vi "Select Device Dialog.vi"(7 "Filter Type":T1=enum."Product Name", 8 "error in (no error)":errorcluster, 10 "Filter Names":string[](array[string]), 11 "Item Ref in":T2 format="%.0x") -> (0 "error out":errorcluster, 1 "Cancelled?":bool, 2 "Selected Alias":string, 3 "Item Ref out":T2=18446744073709551615 format="%.0x")   [LabVIEW 2015, in "NIVS Hardware Discovery.lvlib"]
uses:
  NIVS Hardware Discovery.lvlib
  <vilib>/NI Veristand/Custom Device API/Custom Device Item Ref.ctl
  Types/Filter Type.ctl
  <vilib>/NI Veristand/Custom Device API/Custom Device API.lvlib
panel:
  in  "Cancel":bool
  in  "Use Selected":bool
  in  "Refresh":bool
  in  "Compatible Devices":u16(ring)
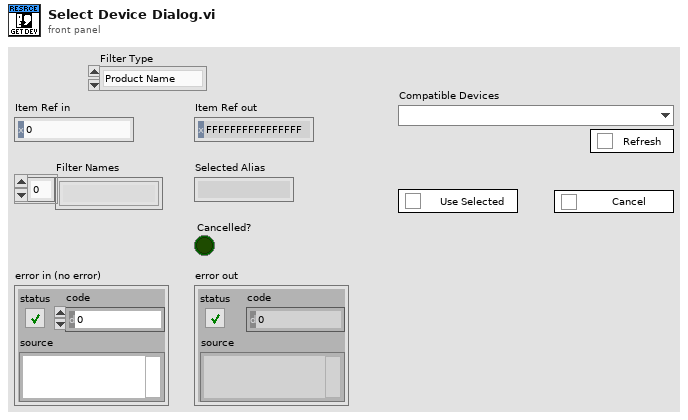
[diagram p1: front panel]
types:
  T1 = typedef "NIVS Hardware Discovery.lvlib/Filter Type.ctl" = enum16{"Device Category", "Product Name", "Ethernet", "XNET", "VISA", "FPGA", "EtherCAT Master", "DAQmx"}
  T2 = typedef "Custom Device API.lvlib/Custom Device Item Ref.ctl" = u64
  T3 = enum32{"Invalid", "Standard", "Closed", "Hidden", "Minimized", "Maximized"}
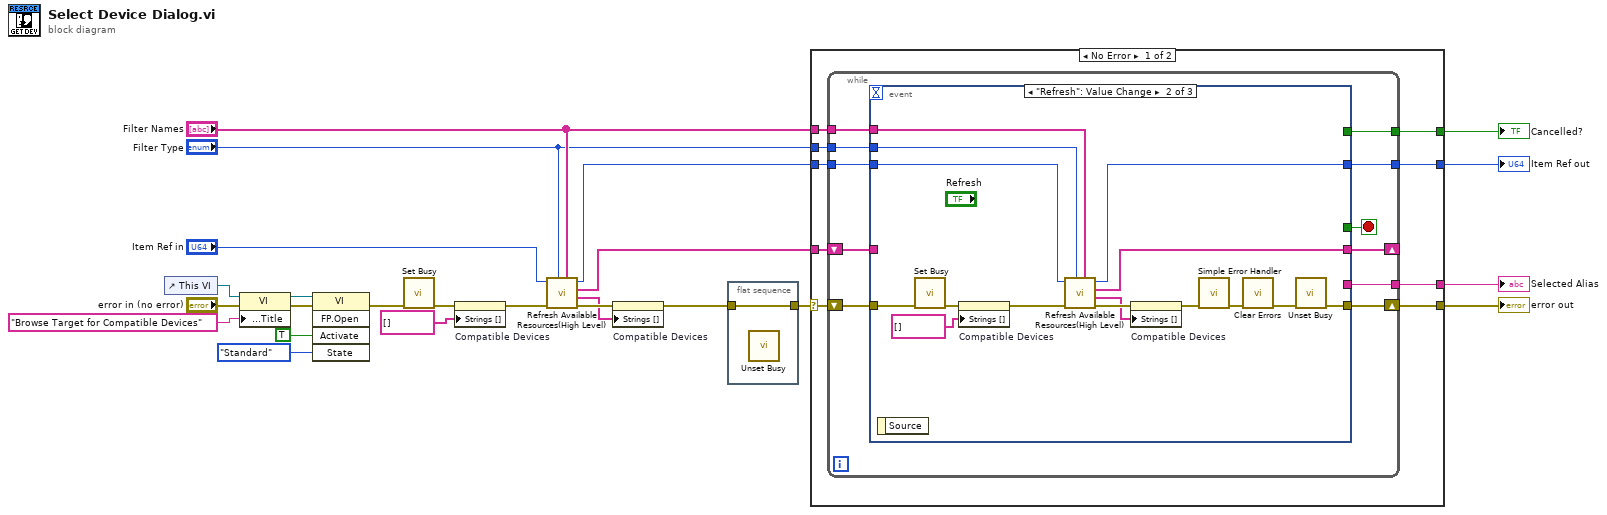
[diagram p0: block diagram]
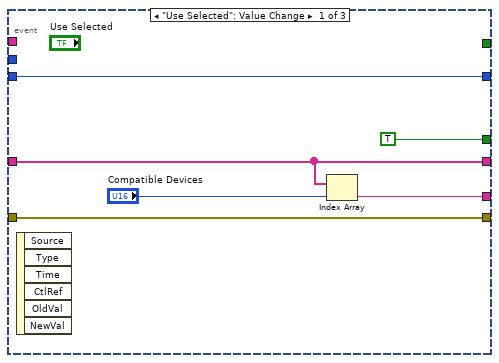
[diagram p2: hidden frame]
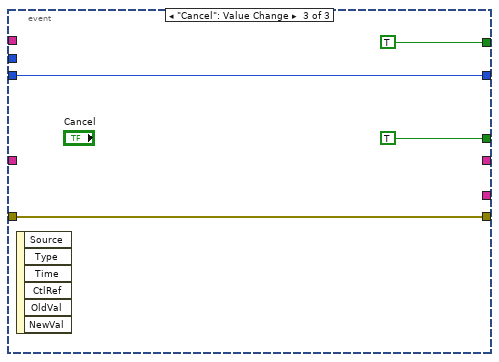
[diagram p3: hidden frame]
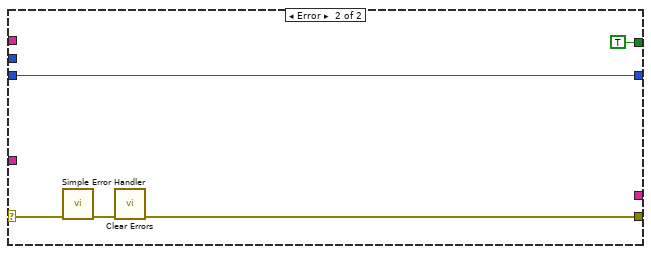
[diagram p4: hidden frame]
diagram:
  n1 = control-ref of="This VI"() -> (w16:refnum<vi>)
  n2 = property class="VI"(reference=w16, error in="error in (no error)", "Front Panel.Title"="Browse Target for Compatible Devices" ("Front Panel Window:Title")) -> (reference out=w14:refnum<vi>, error out=w13:errorcluster)
  n3 = invoke class="VI" method="FP.Open"(reference=w14, error in=w13, "Activate"=TRUE ("Activate?"), "State"=T3."Standard") -> (error out=w4:errorcluster)  [unwired: 1 in, 4 out]
  n4 = call <vilib>:"Set Busy.vi"("error in (no error)"=w4) -> ("error out"=w3:errorcluster)  [unwired: 9 in, 1 out]
  n5 = property on="Compatible Devices" class="Ring (strict)"(error in=w3, "Strings []"=string[] []) -> (error out=w6:errorcluster)  [unwired: 1 in, 1 out]
  n6 = call "Refresh Available Resources(High Level).vi"("Filter Names"="Filter Names", "Filter Type"="Filter Type", "error in (no error)"=w6, "Section Ref in"="Item Ref in") -> ("error out"=w9:errorcluster, "Name and Alias"=w7:string[], "Aliases"=w8:string[], "Section Ref out"=w10:T2)  [unwired: 4 in]
  n7 = property on="Compatible Devices" class="Ring (strict)"(error in=w9, "Strings []"=w7) -> (error out=w1:errorcluster)  [unwired: 1 in, 1 out]
  n8 = flat-sequence {
    tunnel: [w25] -> w2
    tunnel: w1 -> [w25]
    frame #0 {
      n9 = call <vilib>:"Unset Busy.vi"() -> ()  [unwired: 11 in, 1 out]
    }
  }
  n10 = case shown="No Error" w2 {
    selector: w2 -> [w26 w75]
    tunnel: [w34 w72] -> w23
    tunnel: [w33 _] -> w22
    tunnel: "Filter Names" -> [w32 _]
    tunnel: [w31 TRUE] -> w20
    tunnel: [w30 w73] -> w17
    tunnel: "Filter Type" -> [w29 _]
    tunnel: w10 -> [w28 w72]
    tunnel: w8 -> [w27 _]
    frame No Error {
      n11 = while {
        shift-right: [w41] -> w30
        shift-left: w26 -> [w42]
        tunnel: [w44] -> w33
        tunnel: w28 -> [w40]
        shift-right: [w38] -> _
        shift-left: w27 -> [w45]
        tunnel: w32 -> [w39]
        tunnel: [w37] -> w31
        tunnel: [w36] -> w34
        tunnel: w29 -> [w35]
        stop <- w43 stop-if-true
        n12 = event shown="[1] \"Refresh\": Value Change" {
          selector: _ -> [_ _ _]
          dyn-events: _ -> [_ _ _]
          timeout: _ -> [_ _ _]
          tunnel: w45 -> [w47 _ _]
          tunnel: [w50 _ _] -> w44
          tunnel: [TRUE _ TRUE] -> w43
          tunnel: w42 -> [w48 w55 w67]
          tunnel: [w48 w52 w67] -> w41
          tunnel: w40 -> [w46 w66 w68]
          tunnel: w39 -> [_ w62 _]
          tunnel: [w47 w61 _] -> w38
          tunnel: [_ _ TRUE] -> w37
          tunnel: [w46 w65 w68] -> w36
          tunnel: w35 -> [_ w63 _]
          event "Use Selected": Value Change {
            n13 = event-data() -> ()  [unwired: 1 in, 6 out]
            n14 = Index Array(array=w47, index="Compatible Devices") -> (element=w50:string)
          }
          event "Refresh": Value Change {
            n15 = event-data() -> ()  [unwired: 1 in, 1 out]
            n16 = call <vilib>:"Set Busy.vi"("error in (no error)"=w55) -> ("error out"=w54:errorcluster)  [unwired: 9 in, 1 out]
            n17 = property on="Compatible Devices" class="Ring (strict)"(error in=w54, "Strings []"=string[] []) -> (error out=w57:errorcluster)  [unwired: 1 in, 1 out]
            n18 = call "Refresh Available Resources(High Level).vi"("Filter Names"=w62, "Filter Type"=w63, "error in (no error)"=w57, "Section Ref in"=w66) -> ("error out"=w64:errorcluster, "Name and Alias"=w60:string[], "Aliases"=w61:string[], "Section Ref out"=w65:T2)  [unwired: 4 in]
            n19 = property on="Compatible Devices" class="Ring (strict)"(error in=w64, "Strings []"=w60) -> (error out=w58:errorcluster)  [unwired: 1 in, 1 out]
            n20 = call <vilib>:"Simple Error Handler.vi"("error in (no error)"=w58) -> ("error out"=w59:errorcluster)  [unwired: 4 in, 4 out]
            n21 = call <vilib>:"Clear Errors.vi"("error in (no error)"=w59) -> ("error out"=w53:errorcluster)  [unwired: 5 in, 1 out]
            n22 = call <vilib>:"Unset Busy.vi"("error in (no error)"=w53) -> ("error out"=w52:errorcluster)  [unwired: 10 in]
          }
          event "Cancel": Value Change {
            n23 = event-data() -> ()  [unwired: 1 in, 6 out]
          }
        }
      }
    }
    frame Error {
      n24 = call <vilib>:"Simple Error Handler.vi"("error in (no error)"=w75) -> ("error out"=w74:errorcluster)  [unwired: 4 in, 4 out]
      n25 = call <vilib>:"Clear Errors.vi"("error in (no error)"=w74) -> ("error out"=w73:errorcluster)  [unwired: 5 in, 1 out]
    }
  }
  "error out" <- w17
  "Item Ref out" <- w23
  "Selected Alias" <- w22
  "Cancelled?" <- w20
